vi "Autonomous Independent.vi"() -> ()   [LabVIEW 2018]
doc: "This VI is called when autonomous begins, and will automatically be terminated when autonomous ends. You can carry out timed or sensor driven robot movement independently without needing to return to the caller."
uses:
  <vilib>/Rock Robotics/WPI/Utilities/WPI_GetSetVariantRefNum.vi
  <vilib>/Rock Robotics/Network Tables/NT Read String.vi
  MyGlobal.vi
  <vilib>/Rock Robotics/Network Tables/NT Write Numeric Array.vi
panel:
  in  "Mouvements 1 robot centre ecoutille cargo gauche":T1(array[cluster])=[{"Y Joystick Value"=1.0, "Movement Name"="Avance", "X Joystick Value"=0.0, "Temps"=0.65, "R Trigger"=0.5, "L Trigger"=0.0, "Bouton X"=FALSE}, {"Y Joystick Value"=0.0, "Movement Name"="Roues vers la droite", "X Joystick Value"=1.0, "Temps"=0.2, "R Trigger"=0.0, "L Trigger"=0.0, "Bouton X"=FALSE}, {"Y Joystick Value"=0.0, "Movement Name"="Se tasse à droite", "X Joystick Value"=1.0, "Temps"=0.5, "R Trigger"=0.5, "L Trigger"=0.0, "Bouton X"=FALSE}, {"Y Joystick Value"=1.0, "Movement Name"="roues vers l'avant", "X Joystick Value"=0.0, "Temps"=0.2, "R Trigger"=0.0, "L Trigger"=0.0, "Bouton X"=FALSE}, {"Y Joystick Value"=1.0, "Movement Name"="Avance", "X Joystick Value"=0.0, "Temps"=0.5, "R Trigger"=0.5, "L Trigger"=0.0, "Bouton X"=FALSE}, {"Y Joystick Value"=0.0, "Movement Name"="Relâche le disque", "X Joystick Value"=0.0, "Temps"=1.5, "R Trigger"=0.0, "L Trigger"=0.0, "Bouton X"=TRUE}, {"Y Joystick Value"=1.0, "Movement Name"="Recule", "X Joystick Value"=0.0, "Temps"=0.5, "R Trigger"=0.0, "L Trigger"=0.5, "Bouton X"=TRUE}]
  in  "Mouvements 1 robot droite ecoutille cargo droite":T1(array[cluster])=[{"Y Joystick Value"=1.0, "Movement Name"="Avance", "X Joystick Value"=0.0, "Temps"=0.65, "R Trigger"=0.5, "L Trigger"=0.0, "Bouton X"=FALSE}, {"Y Joystick Value"=0.0, "Movement Name"="Roues vers la gauche", "X Joystick Value"=-1.0, "Temps"=0.2, "R Trigger"=0.0, "L Trigger"=0.0, "Bouton X"=FALSE}, {"Y Joystick Value"=0.0, "Movement Name"="Se tasse à gauche", "X Joystick Value"=-1.0, "Temps"=0.5, "R Trigger"=0.5, "L Trigger"=0.0, "Bouton X"=FALSE}, {"Y Joystick Value"=1.0, "Movement Name"="roues vers l'avant", "X Joystick Value"=0.0, "Temps"=0.2, "R Trigger"=0.0, "L Trigger"=0.0, "Bouton X"=FALSE}, {"Y Joystick Value"=1.0, "Movement Name"="Avance", "X Joystick Value"=0.0, "Temps"=0.5, "R Trigger"=0.5, "L Trigger"=0.0, "Bouton X"=FALSE}, {"Y Joystick Value"=0.0, "Movement Name"="Relâche le disque", "X Joystick Value"=0.0, "Temps"=1.5, "R Trigger"=0.0, "L Trigger"=0.0, "Bouton X"=TRUE}, {"Y Joystick Value"=1.0, "Movement Name"="Recule", "X Joystick Value"=0.0, "Temps"=0.5, "R Trigger"=0.0, "L Trigger"=0.5, "Bouton X"=TRUE}]
  in  "Mouvements 1 robot gauche ecoutille cargo gauche":T1(array[cluster])=[{"Y Joystick Value"=1.0, "Movement Name"="Avance", "X Joystick Value"=0.0, "Temps"=0.65, "R Trigger"=0.5, "L Trigger"=0.0, "Bouton X"=FALSE}, {"Y Joystick Value"=0.0, "Movement Name"="Roues vers la droite", "X Joystick Value"=1.0, "Temps"=0.2, "R Trigger"=0.0, "L Trigger"=0.0, "Bouton X"=FALSE}, {"Y Joystick Value"=0.0, "Movement Name"="Se tasse à droite", "X Joystick Value"=1.0, "Temps"=0.5, "R Trigger"=0.5, "L Trigger"=0.0, "Bouton X"=FALSE}, {"Y Joystick Value"=1.0, "Movement Name"="roues vers l'avant", "X Joystick Value"=0.0, "Temps"=0.2, "R Trigger"=0.0, "L Trigger"=0.0, "Bouton X"=FALSE}, {"Y Joystick Value"=1.0, "Movement Name"="Avance", "X Joystick Value"=0.0, "Temps"=0.5, "R Trigger"=0.5, "L Trigger"=0.0, "Bouton X"=FALSE}, {"Y Joystick Value"=0.0, "Movement Name"="Relâche le disque", "X Joystick Value"=0.0, "Temps"=1.5, "R Trigger"=0.0, "L Trigger"=0.0, "Bouton X"=TRUE}, {"Y Joystick Value"=1.0, "Movement Name"="Recule", "X Joystick Value"=0.0, "Temps"=0.5, "R Trigger"=0.0, "L Trigger"=0.5, "Bouton X"=TRUE}]
  # "TESTER LES DISTANCES / TIMINGS pour chaque séquence"
  # "(distance+3.1052)/66.526=temps"
  # "avance a la balance et tourne pour ~39 pouces"
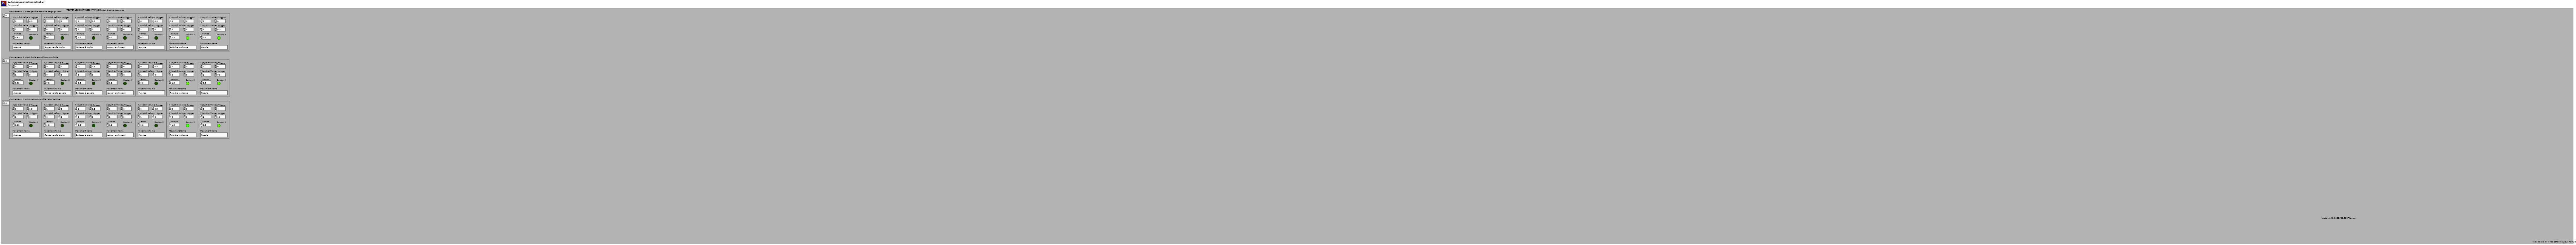
[diagram p1: front panel]
types:
  T1 = cluster{"Y Joystick Value":dbl, "Movement Name":string, "X Joystick Value":dbl, "Temps":dbl, "R Trigger":dbl, "L Trigger":dbl, "Bouton X":bool}[]
  T2 = typedef "WPI_JoystickDevRef.ctl" = cluster{"Device":T3}
  T3 = typedef "WPI_JoystickDeviceEnum.ctl" = enum16{"USB 0", "USB 1", "USB 2", "USB 3", "USB 4", "USB 5"}
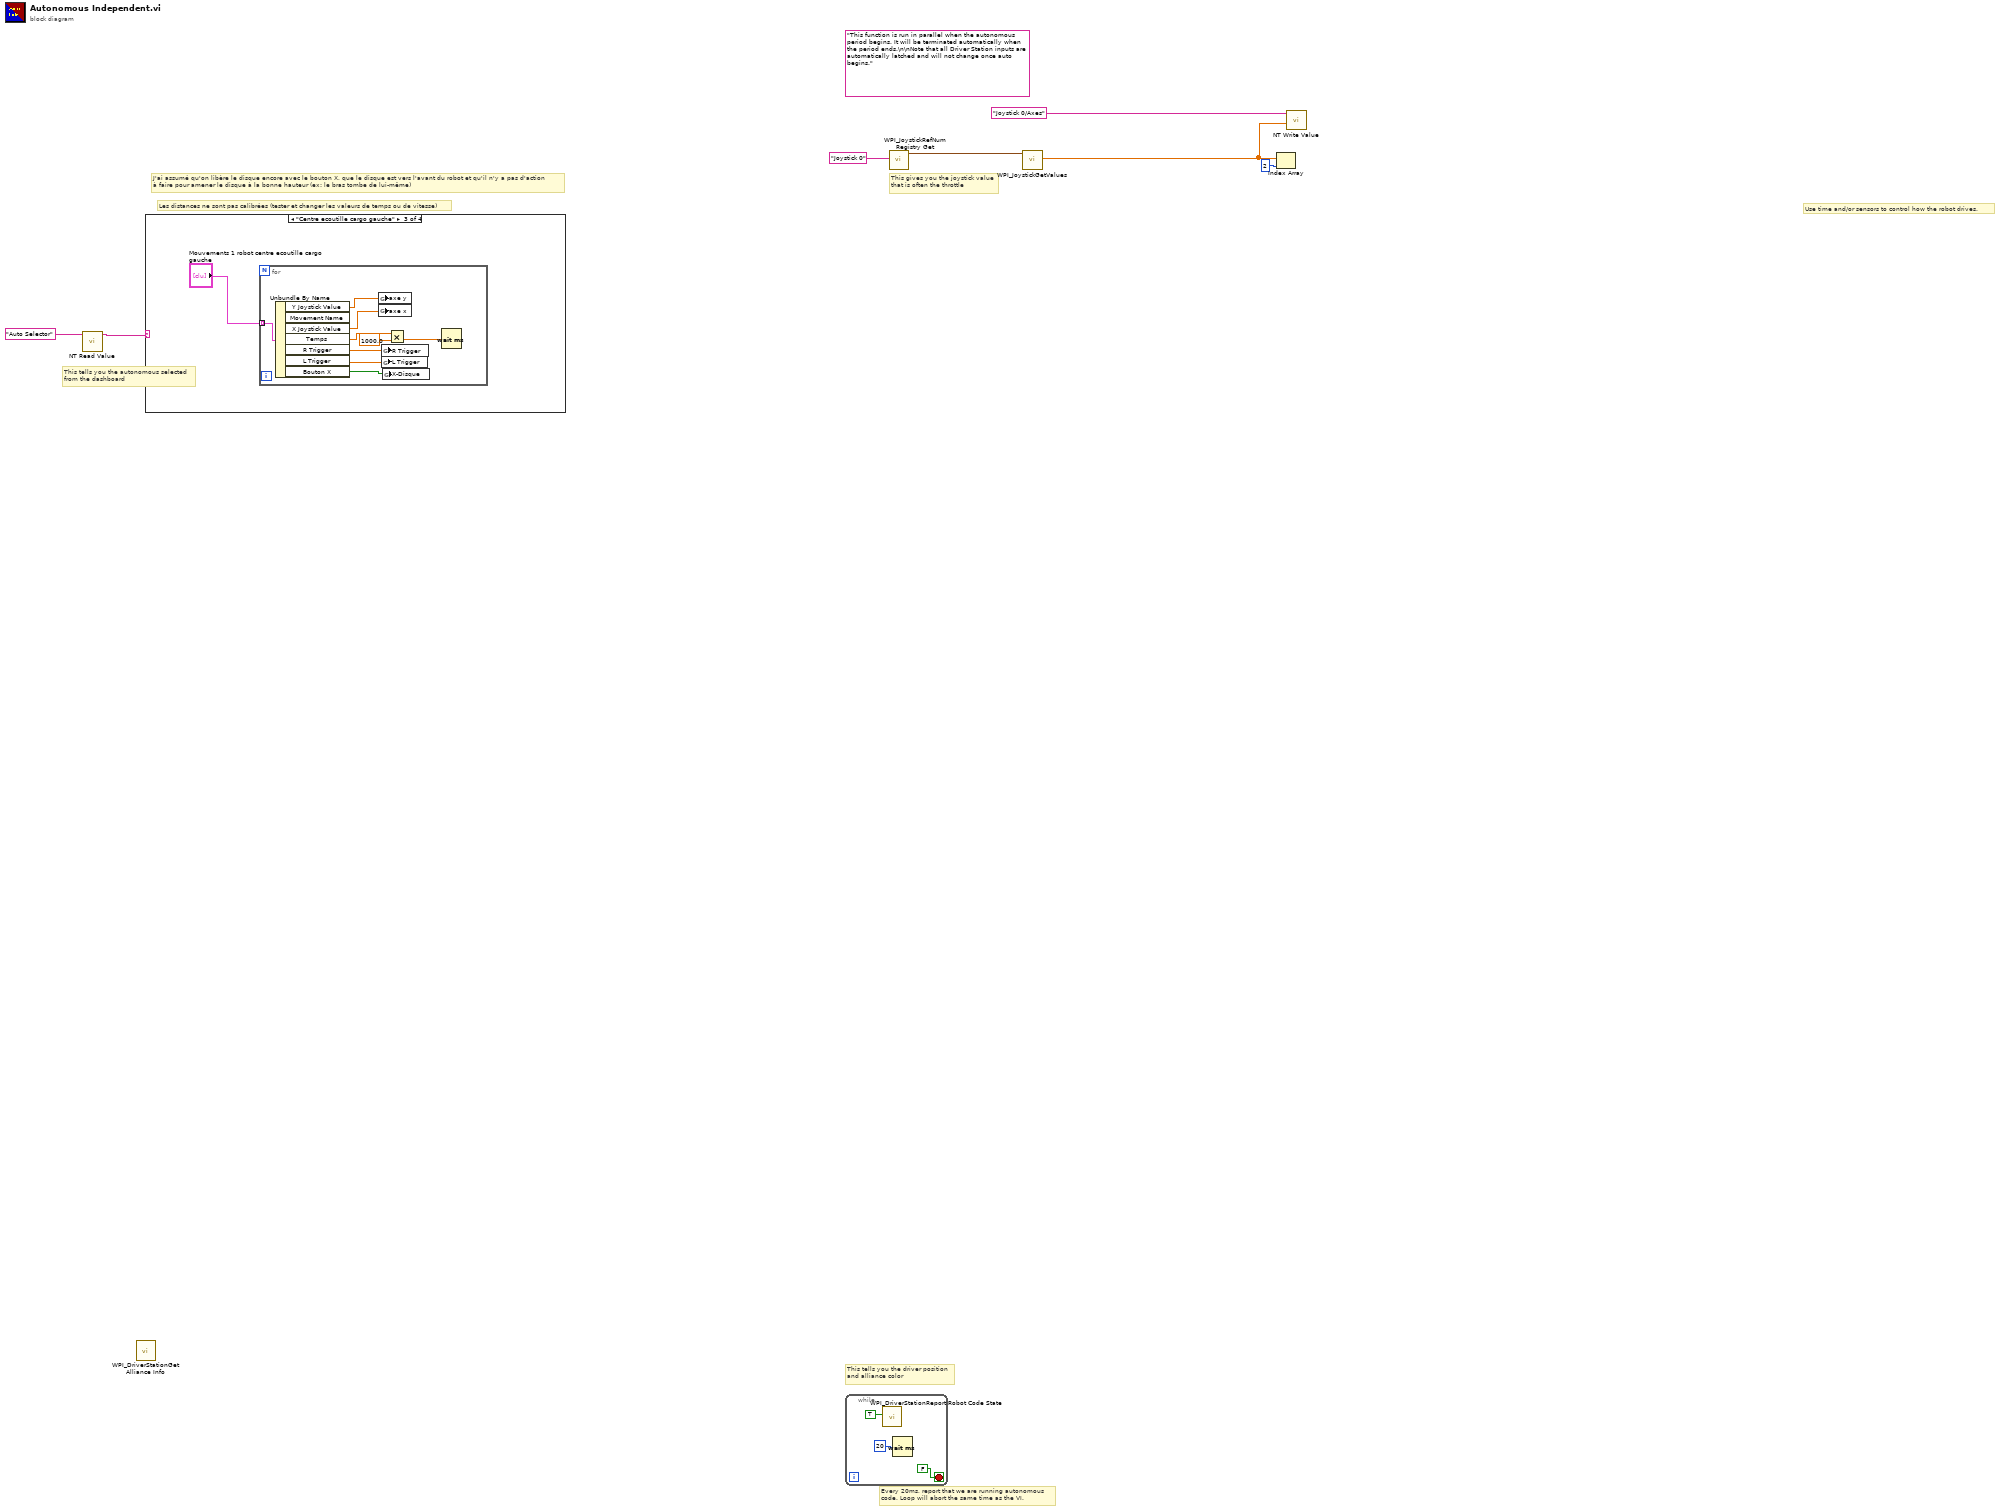
[diagram p0: block diagram]
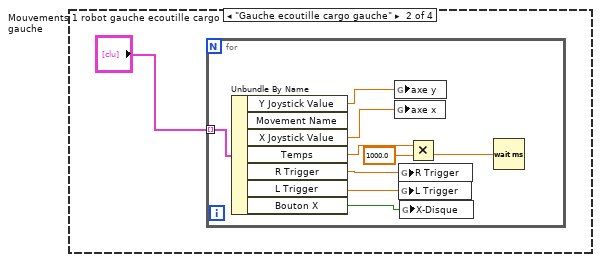
[diagram p3: hidden frame]
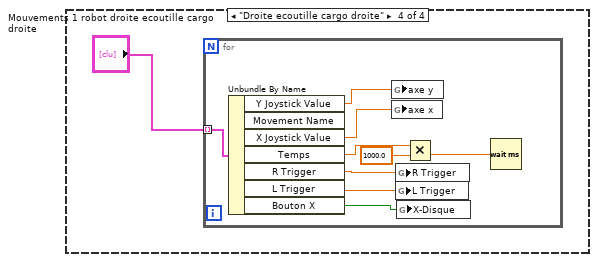
[diagram p4: hidden frame]
diagram:
  (unwired) "This function is run in parallel when the autonomous period begins. It will be terminated automatically when the period ends.\n\nNote that all Driver Station inputs are automatically latched and will not change once auto begins."
  # "Les distances ne sont pas calibrées (tester et changer les valeurs de temps ou de vitesse)"
  # "J'ai assumé qu'on libère le disque encore avec le bouton X, que le disque est vers l'avant du robot et qu'il n'y a pas d'action \nà faire pour amener le disque à la bonne hauteur (ex: le bras tombe de lui-même)"
  # "This tells you the autonomous selected\nfrom the dashboard"
  # "This gives you the joystick value\nthat is often the throttle"
  # "Every 20ms, report that we are running autonomous\ncode. Loop will abort the same time as the VI."
  # "Use time and/or sensors to control how the robot drives."
  # "This tells you the driver position\nand alliance color"
  n1 = call-poly <vilib>:"NT Read Value.vi"("Name"="Auto Selector") -> ("String"=w3:string)  [unwired: 9 in, 1 out]
  n2 = call <vilib>:"WPI_DriverStationGet Alliance Info.vi"() -> ()  [unwired: 12 out]
  n3 = case shown="\"Centre ecoutille cargo gauche\"" w3 {
    frame Default {
    }
    frame "Gauche ecoutille cargo gauche" {
      n4 = for {
        tunnel: "Mouvements 1 robot gauche ecoutille cargo gauche" -> [w17] mode=indexing
        n5 = Unbundle By Name(w17) -> ("Y Joystick Value"=w15:dbl, "X Joystick Value"=w16:dbl, "Temps"=w14:dbl, "R Trigger"=w11:dbl, "L Trigger"=w10:dbl, "Bouton X"=w9:bool)  [unwired: 1 out]
        n6 = global write "MyGlobal.vi" "axe y"(w15) -> ()
        n7 = global write "MyGlobal.vi" "axe x"(w16) -> ()
        n8 = global write "MyGlobal.vi" "R Trigger"(w11) -> ()
        n9 = global write "MyGlobal.vi" "L Trigger"(w10) -> ()
        n10 = global write "MyGlobal.vi" "X-Disque"(w9) -> ()
        n11 = Multiply(x=w14, y=1000.0) -> (x*y=w13:dbl)
        n12 = Wait (ms)(milliseconds to wait=w13) -> ()  [unwired: 1 out]
      }
    }
    frame "Centre ecoutille cargo gauche" {
      n13 = for {
        tunnel: "Mouvements 1 robot centre ecoutille cargo gauche" -> [w27] mode=indexing
        n14 = Unbundle By Name(w27) -> ("Y Joystick Value"=w25:dbl, "X Joystick Value"=w26:dbl, "Temps"=w24:dbl, "R Trigger"=w21:dbl, "L Trigger"=w20:dbl, "Bouton X"=w19:bool)  [unwired: 1 out]
        n15 = global write "MyGlobal.vi" "axe y"(w25) -> ()
        n16 = global write "MyGlobal.vi" "axe x"(w26) -> ()
        n17 = global write "MyGlobal.vi" "R Trigger"(w21) -> ()
        n18 = global write "MyGlobal.vi" "L Trigger"(w20) -> ()
        n19 = global write "MyGlobal.vi" "X-Disque"(w19) -> ()
        n20 = Multiply(x=w24, y=1000.0) -> (x*y=w23:dbl)
        n21 = Wait (ms)(milliseconds to wait=w23) -> ()  [unwired: 1 out]
      }
    }
    frame "Droite ecoutille cargo droite" {
      n22 = for {
        tunnel: "Mouvements 1 robot droite ecoutille cargo droite" -> [w37] mode=indexing
        n23 = Unbundle By Name(w37) -> ("Y Joystick Value"=w35:dbl, "X Joystick Value"=w36:dbl, "Temps"=w34:dbl, "R Trigger"=w31:dbl, "L Trigger"=w30:dbl, "Bouton X"=w29:bool)  [unwired: 1 out]
        n24 = global write "MyGlobal.vi" "axe y"(w35) -> ()
        n25 = global write "MyGlobal.vi" "axe x"(w36) -> ()
        n26 = global write "MyGlobal.vi" "R Trigger"(w31) -> ()
        n27 = global write "MyGlobal.vi" "L Trigger"(w30) -> ()
        n28 = global write "MyGlobal.vi" "X-Disque"(w29) -> ()
        n29 = Multiply(x=w34, y=1000.0) -> (x*y=w33:dbl)
        n30 = Wait (ms)(milliseconds to wait=w33) -> ()  [unwired: 1 out]
      }
    }
  }
  n31 = while {
    stop <- FALSE stop-if-true
    n32 = call <vilib>:"WPI_DriverStationReport Robot Code State.vi"("Autonomous"=TRUE) -> ()  [unwired: 10 in, 1 out]
    n33 = Wait (ms)(milliseconds to wait=u32 20) -> ()  [unwired: 1 out]
  }
  n34 = call <vilib>:"WPI_JoystickRefNum Registry Get.vi"("refnum name"="Joystick 0") -> ("JoystickDevRef"=w6:T2)  [unwired: 1 in, 9 out]
  n35 = call <vilib>:"WPI_JoystickGetValues.vi"("JoystickDevRef"=w6) -> ("Axes"=w2:dbl[])  [unwired: 6 in, 4 out]
  n36 = Index Array(array=w2, index=2) -> ()  [unwired: 1 out]
  n37 = call-poly <vilib>:"NT Write Value.vi"("Numeric Array"=w2, "Name"="Joystick 0/Axes") -> ()  [unwired: 9 in, 1 out]
